vi "Channel Power Enable.vi"(7 "All Channels (F)":bool, 8 "error in (no error)":errorcluster, 9 "Enable (OFF)":bool, 10 "Channel (0)":u8, 11 "BoardHandle":T1) -> (0 "error out":errorcluster, 3 "BoardHandle out":T1)   [LabVIEW 2018, in "CAEN PSM.lvlib"]
doc: "Enables or disables the output of the power supply."
uses:
  <instrlib>/CAEN PSM/CAEN PSM.lvlib
  <instrlib>/CAEN PSM/Private/BoardHandle.ctl
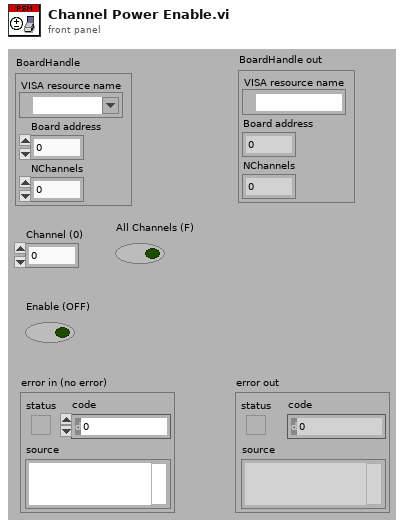
[diagram p1: front panel]
types:
  T1 = typedef "CAEN PSM.lvlib/BoardHandle.ctl" = cluster{"VISA resource name":refnum<visa-resource-name>, "Board address":u8, "NChannels":u8}
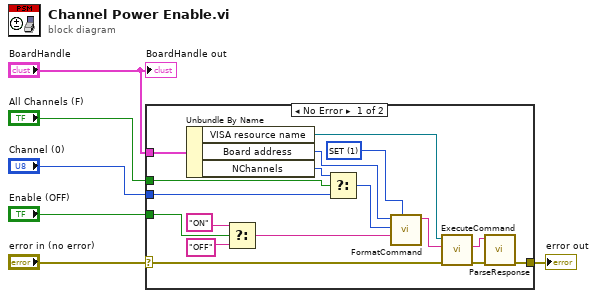
[diagram p0: block diagram]
diagram:
  n1 = case shown="No Error" "error in (no error)" {
    selector: "error in (no error)" -> [w7 w24]
    tunnel: "Enable (OFF)" -> [w22 _]
    tunnel: "All Channels (F)" -> [w17 _]
    tunnel: "Channel (0)" -> [w15 _]
    tunnel: [w10 w24] -> w3
    tunnel: "BoardHandle" -> [w8 _]
    frame No Error {
      w18 = u8 1 items=["MON", "SET"] ("CMD")
      n2 = Unbundle By Name(w8) -> ("VISA resource name"=w13:refnum<visa-resource-name>, "Board address"=w23:u8, "NChannels"=w16:u8)
      n3 = Select(t="ON", s=w22, f="OFF") -> (s? t:f=w19:string)
      n4 = Select(t=w16, s=w17, f=w15) -> (s? t:f=w14:u8)
      n5 = call <instrlib>:"FormatCommand.vi"("CMD (MON)"=w18, "PAR"=w19, "CH"=w14, "BD (0)"=w23) -> ("cmd"=w12:string)  [unwired: 7 in]
      n6 = call <instrlib>:"ExecuteCommand.vi"("error in (no error)"=w7, "Command"=w12, "VISA resource name"=w13) -> ("error out"=w11:errorcluster, "Response"=w9:string)  [unwired: 6 in, 1 out]
      n7 = call <instrlib>:"ParseResponse.vi"("error in (no error)"=w11, "Response"=w9) -> ("error out"=w10:errorcluster)  [unwired: 6 in, 3 out]
    }
    frame Error {
    }
  }
  "error out" <- w3
  "BoardHandle out" <- "BoardHandle"
